vi "DigitalDisplayVisible.vi"(6 "error in":errorcluster, 9 "Slide in":refnum<class "Slide.lvclass">) -> (0 "error out":errorcluster, 3 "Slide out":refnum<class "Slide.lvclass">, 4 "digital display":bool)   [LabVIEW 2014, in "Slide.lvclass"]
uses:
  Slide.lvclass
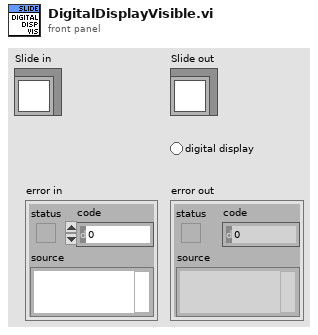
[diagram p1: front panel]
types:
  T1 = typedef "LVRectTypeDef.ctl" = cluster{"Left":i16, "Top":i16, "Right":i16, "Bottom":i16}
  T2 = cluster{"left":i16, "top":i16, "right":i16, "bottom":i16}
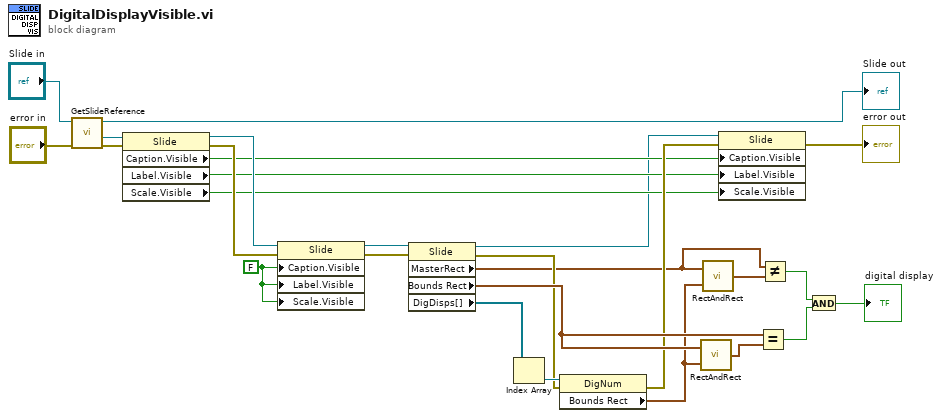
[diagram p0: block diagram]
diagram:
  w10 = FALSE ("Caption.Visible")
  n1 = call "GetSlideReference.vi"("error in"="error in", "Slide in"="Slide in") -> ("error out"=w4:errorcluster, "slide reference"=w5:refnum<vi>, "Slide out"=→"Slide out":refnum<class "Slide.lvclass">)  [unwired: 7 in]
  n2 = property class="Slide"(reference=w5, error in=w4) -> (reference out=w19:refnum<vi>, error out=w18:errorcluster, "Caption.Visible"=w13:bool, "Label.Visible"=w12:bool, "Scale.Visible"=w11:bool)
  n3 = property class="Slide"(reference=w19, error in=w18, "Caption.Visible"=w10, "Label.Visible"=w10, "Scale.Visible"=w10) -> (reference out=w17:refnum<vi>, error out=w16:errorcluster)
  n4 = property class="Slide"(reference=w17, error in=w16) -> (reference out=w9:refnum<vi>, error out=w15:errorcluster, "MasterRect"=w8:T1, "Bounds Rect"=w22:T1, "DigDisps[]"=w25:refnum<vi>[])
  n5 = Index Array(array=w25) -> (element=w24:refnum<vi>)  [unwired: 1 in]
  n6 = property class="DigNum"(reference=w24, error in=w15) -> (error out=w14:errorcluster, "Bounds Rect"=w21:T1)  [unwired: 1 out]
  n7 = call <vilib>:"RectAndRect.vi"("rect b"=w21, "rect a"=w22) -> ("union rect"=w23:T2)
  n8 = call <vilib>:"RectAndRect.vi"("rect b"=w21, "rect a"=w8) -> ("union rect"=w20:T2)
  n9 = property class="Slide"(reference=w9, error in=w14, "Caption.Visible"=w13, "Label.Visible"=w12, "Scale.Visible"=w11) -> (error out=→"error out":errorcluster)  [unwired: 1 out]
  n10 = Equal?(x=w22, y=w23) -> (x = y?=w6:bool)
  n11 = Not Equal?(x=w8, y=w20) -> (x != y?=w7:bool)
  n12 = And(x=w7, y=w6) -> (x .and. y?=→"digital display":bool)
